vi "berry.vi"() -> ()   [LabVIEW 2018]
panel:
  in  "D":bool
  in  "C":bool
  in  "B":bool
  in  "A":bool
  out "Boolean 6":bool
  out "Boolean 5":bool
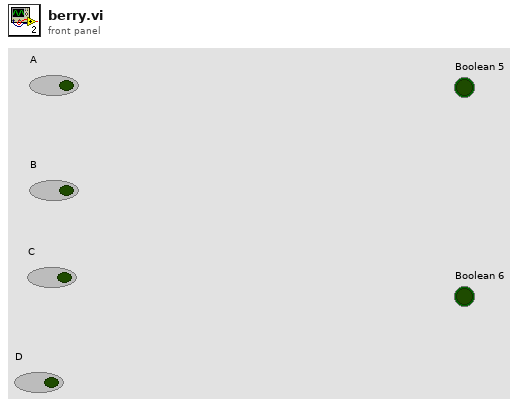
[diagram p1: front panel]
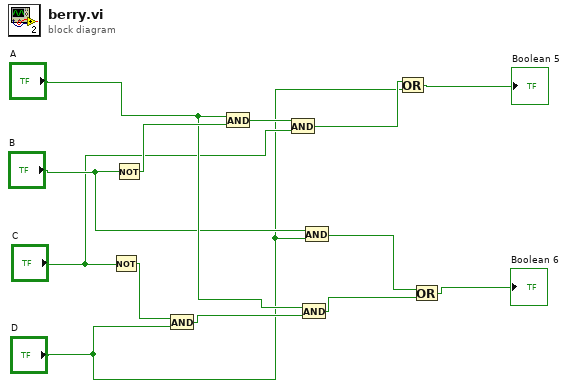
[diagram p0: block diagram]
diagram:
  n1 = Not(x="C") -> (.not. x?=w11:bool)
  n2 = Not(x="B") -> (.not. x?=w13:bool)
  n3 = And(x=w11, y="D") -> (x .and. y?=w10:bool)
  n4 = And(x="A", y=w13) -> (x .and. y?=w12:bool)
  n5 = And(x=w12, y="C") -> (x .and. y?=w7:bool)
  n6 = And(x="A", y=w10) -> (x .and. y?=w8:bool)
  n7 = And(x="B", y="D") -> (x .and. y?=w9:bool)
  n8 = Or(x=w7, y="D") -> (x .or. y?=→"Boolean 5":bool)
  n9 = Or(x=w9, y=w8) -> (x .or. y?=→"Boolean 6":bool)
